vi "Bounce Window_Log In.vi"(8 "Error in":errorcluster, 11 "User Account Table Path":path) -> (0 "Error Out":errorcluster, 3 "User Account Data Out":T1={"帳號 :"="", "權限等級："=enum."開發人員", "建立時間："="", "修改時間："="", "到期時間："="", "狀態："=enum."可使用", "期限："=enum."一天", "密碼："=""})   [LabVIEW 2015]
uses:
  <vilib>/Utility/miscctls.llb/LVPointTypeDef.ctl
panel:
  in  "取消":bool
  in  "登入":bool
  in  "密碼 :":string
  in  "帳號 :":string
  # "帳號登入"
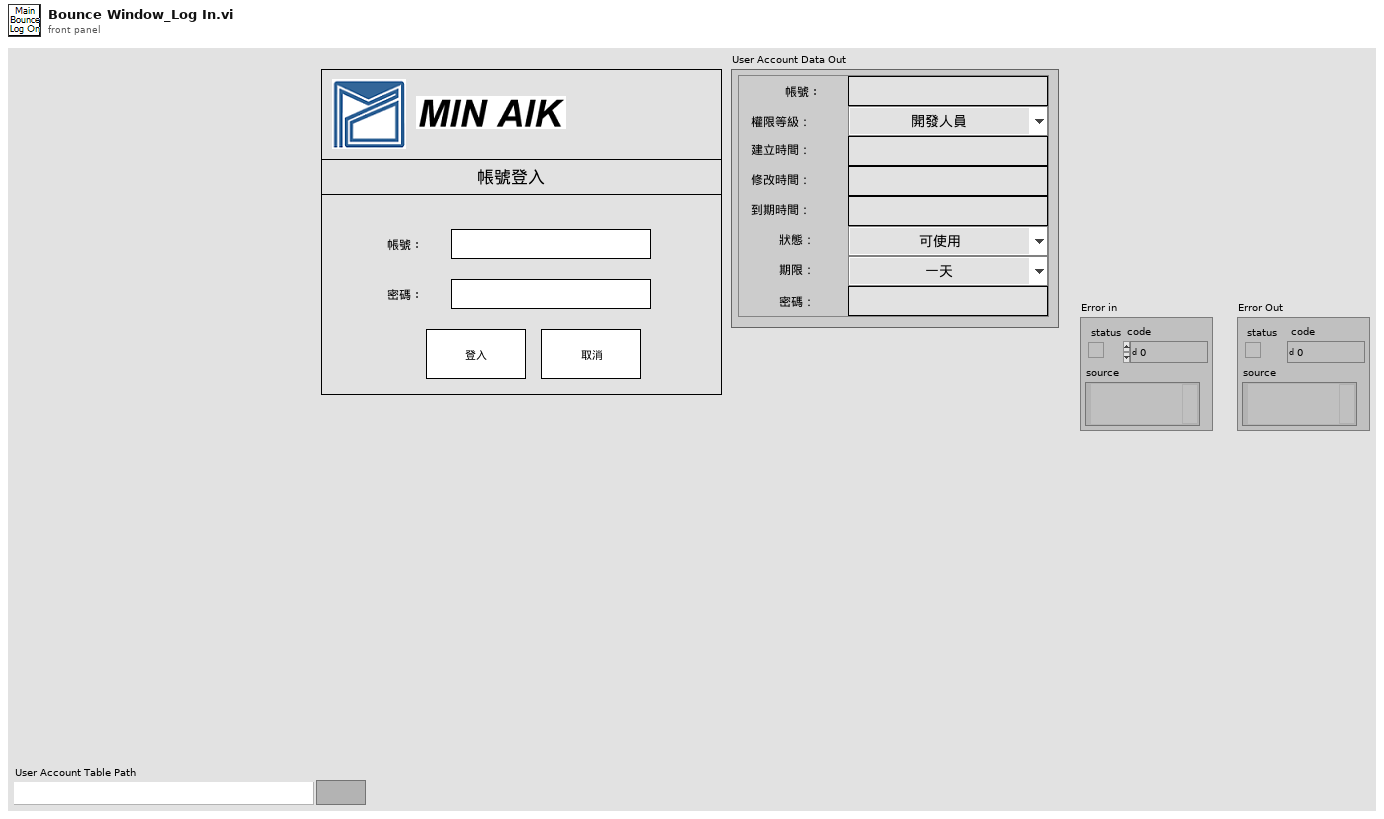
[diagram p1: front panel]
types:
  T1 = typedef "Control_User account_Data.ctl" = cluster{"帳號 :":string, "權限等級：":T2, "建立時間：":string, "修改時間：":string, "到期時間：":string, "狀態：":T3, "期限：":T4, "密碼：":string}
  T2 = typedef "Control_User account_Permissions.ctl" = enum16{"開發人員", "管理者", "工程師", "作業員"}
  T3 = typedef "Control_User Accounts_Status.ctl" = enum16{"可使用", "不可使用"}
  T4 = typedef "Control_User account_Date.ctl" = enum16{"零天", "一天", "七天", "一個月", "一年", "三年"}
  T5 = typedef "Control_Bounce Window_User Accounts_Data Action" = enum16{"Initialize", "Set Data", "Set Data Array", "Replace Data", "Delete Data", "Get Data", "Get Data Array"}
  T6 = typedef "LVPointTypeDef.ctl" = cluster{"Horizontal":i16, "Vertical":i16}
  T7 = typedef "eventvkey.ctl" = enum16{"ASCII", "Enter", "Return", "Shift", "Ctrl", "Alt", "Cmd", "Opt", "Caps", "NumLock", "Clear", "Break", "Up", "Down", "Left", "Right", "Insert", "Delete", "Home", "End", "PageUp", "PageDown", "Escape", "Help", "Pause", "ScrollLock", "F1", "F2", "F3", "F4", "F5", "F6", "F7", "F8", "F9", "F10", "F11", "F12", "F13", "F14", "F15", "F16", "F17", "F18", "F19", "F20", "F21", "F22", "F23", "F24", "Play", "VolumeUp", "VolumeDown", "Mute", "Two Byte Char"}
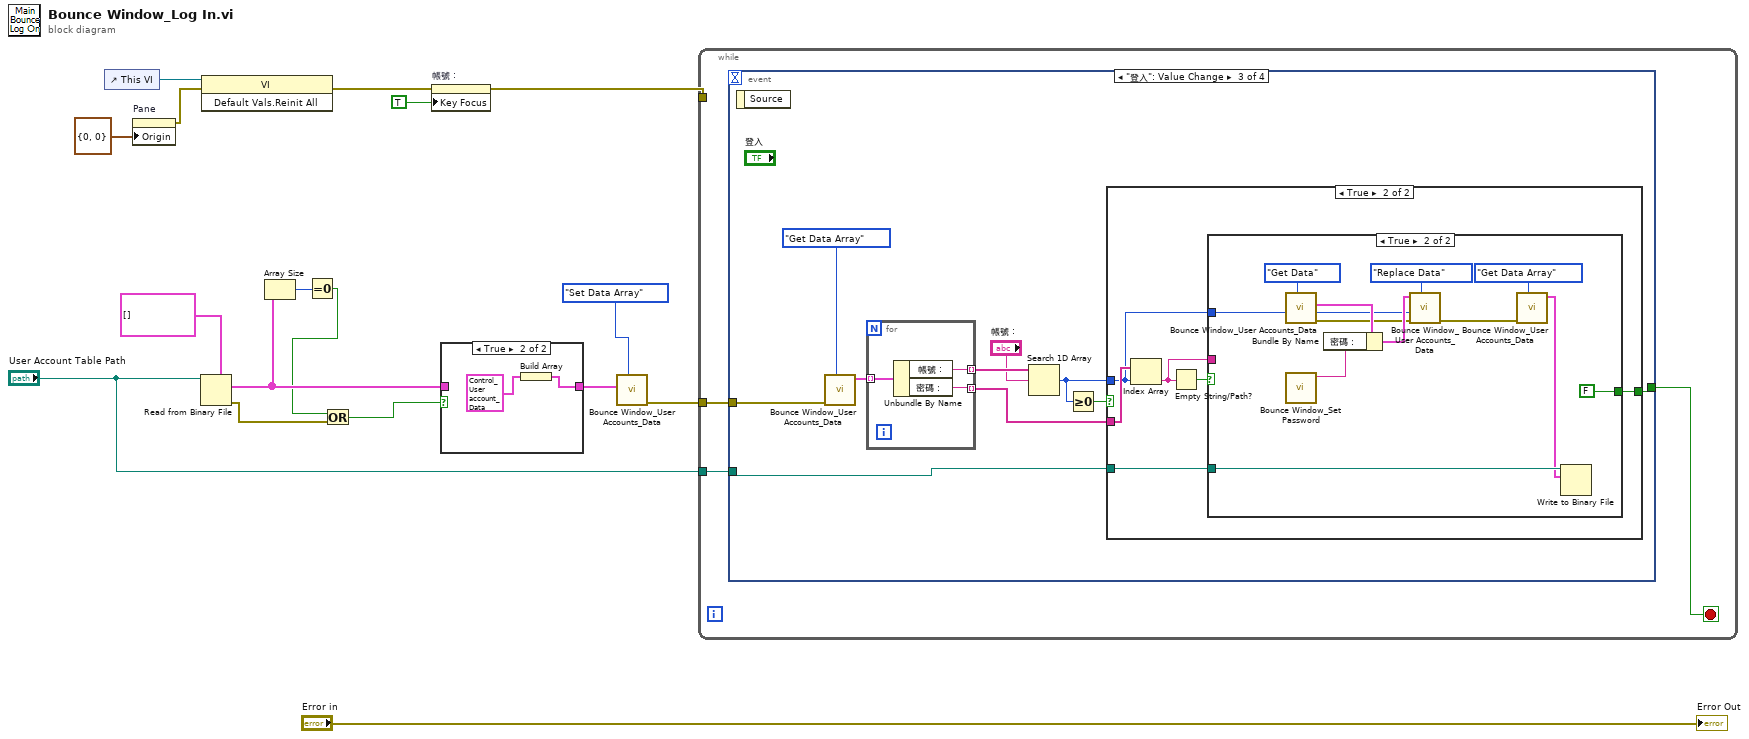
[diagram p0: block diagram]
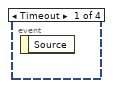
[diagram p3: hidden frame]
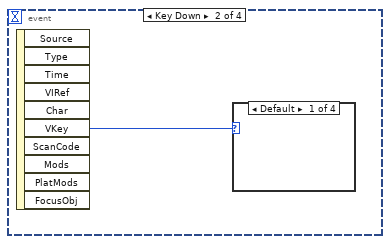
[diagram p4: hidden frame]
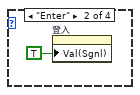
[diagram p5: hidden frame]
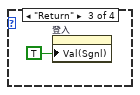
[diagram p6: hidden frame]
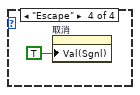
[diagram p7: hidden frame]
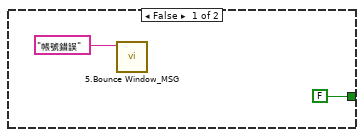
[diagram p8: hidden frame]
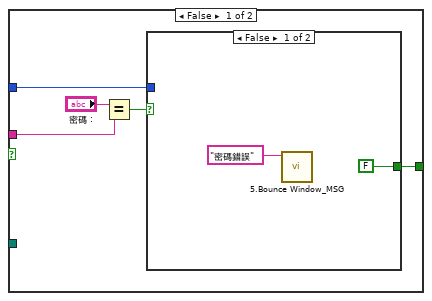
[diagram p9: hidden frame]
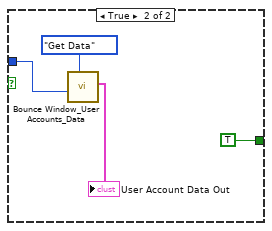
[diagram p10: hidden frame]
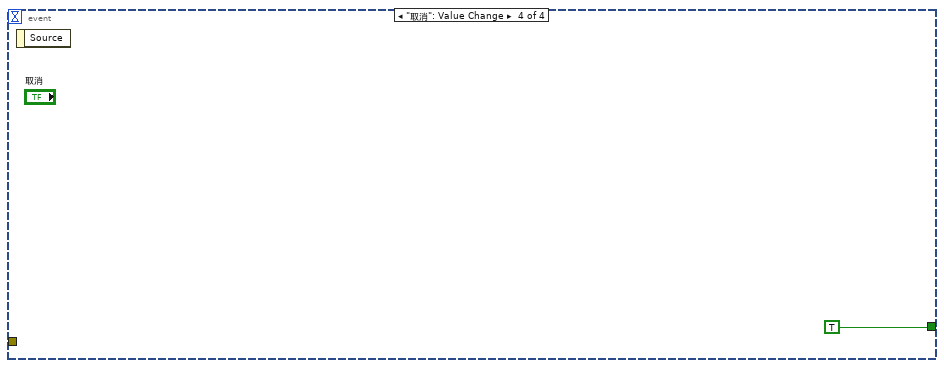
[diagram p11: hidden frame]
diagram:
  n1 = control-ref of="This VI"() -> (w9:refnum<vi>)
  n2 = property on="Pane" class="Pane"("Origin"=T6 {"Horizontal"=0, "Vertical"=0}) -> (error out=w8:errorcluster)  [unwired: 2 in, 1 out]
  n3 = Read from Binary File(5:T1[] [], 11:"User Account Table Path") -> (0:w2:errorcluster, 2:w5:T1[])  [unwired: 4 in, 2 out]
  n4 = invoke class="VI" method="Default Vals.Reinit All"(reference=w9, error in=w8) -> (error out=w11:errorcluster)  [unwired: 1 in, 2 out]
  n5 = Array Size(array=w5) -> (size(s)=w4:i32)
  n6 = Equal To 0?(x=w4) -> (x = 0?=w3:bool)
  n7 = Or(x=w3, y=w2) -> (x .or. y?=w1:bool)
  n8 = property on="帳號 :" class="Str"(error in=w11, "Key Focus"=TRUE) -> (error out=w10:errorcluster)  [unwired: 1 in, 1 out]
  n9 = case shown="True" w1 {
    tunnel: w5 -> [w18 _]
    tunnel: [w18 w19] -> w7
    frame False {
    }
    frame True {
      n10 = Build Array(T1 {"帳號 :"="admin", "權限等級："=enum."開發人員", "建立時間："="2000/01/01", "修改時間："="", "到期時間："="9999/12/31", "狀態："=enum."可使用", "期限："=enum."三年", "密碼："="1234"} ("User Account Data")) -> (w19:T1[])
    }
  }
  n11 = call "Bounce Window_User Accounts_Data.vi"("Table_Action"=Control_Bounce_Window_User_Accounts_Data_Action."Set Data Array", "Data Array In"=w7) -> ("Error Out"=w13:errorcluster)  [unwired: 7 in, 2 out]
  n12 = while {
    tunnel: "User Account Table Path" -> [w22]
    tunnel: w13 -> [w21]
    tunnel: w10 -> [_]
    stop <- w23 stop-if-true
    n13 = event shown="[2] \"登入\": Value Change" {
      selector: _ -> [_ _ _ _]
      dyn-events: _ -> [_ _ _ _]
      timeout: _ -> [_ _ _ _]
      tunnel: [_ _ w32 TRUE] -> w23
      tunnel: w22 -> [_ _ w31 _]
      tunnel: w21 -> [_ _ w28 _]
      event Timeout {
        n14 = event-data() -> ()  [unwired: 1 in, 1 out]
      }
      event Key Down {
        n15 = event-data() -> ("VKey"=w24:T7)  [unwired: 1 in, 9 out]
        n16 = case shown="Default" w24 {
          frame Default {
          }
          frame "Enter" {
            n17 = property on="登入" class="Bool (strict)"("Val(Sgnl)"=TRUE ("Value (Signaling)")) -> ()  [unwired: 2 in, 2 out]
          }
          frame "Return" {
            n18 = property on="登入" class="Bool (strict)"("Val(Sgnl)"=TRUE ("Value (Signaling)")) -> ()  [unwired: 2 in, 2 out]
          }
          frame "Escape" {
            n19 = property on="取消" class="Bool (strict)"("Val(Sgnl)"=TRUE ("Value (Signaling)")) -> ()  [unwired: 2 in, 2 out]
          }
        }
      }
      event "登入": Value Change {
        n20 = event-data() -> ()  [unwired: 1 in, 1 out]
        n21 = call "Bounce Window_User Accounts_Data.vi"("Table_Action"=Control_Bounce_Window_User_Accounts_Data_Action."Get Data Array", "Error in"=w28) -> ("Data Array Out"=w29:T1[])  [unwired: 7 in, 2 out]
        n22 = for {
          tunnel: w29 -> [w71] mode=indexing
          tunnel: [w70] -> w37 mode=indexing
          tunnel: [w69] -> w33 mode=indexing
          n23 = Unbundle By Name(w71) -> ("帳號 :"=w70:string, "密碼："=w69:string)
        }
        n24 = Search 1D Array(1D array=w37, element="帳號 :") -> (index of element=w34:i32)  [unwired: 1 in]
        n25 = Greater Or Equal To 0?(x=w34) -> (x >= 0?=w35:bool)
        n26 = case shown="True" w35 {
          tunnel: w34 -> [_ w41]
          tunnel: w33 -> [_ w45]
          tunnel: [FALSE w42] -> w32
          tunnel: w31 -> [_ w40]
          frame False {
            n27 = call "5.Bounce Window_MSG.vi"("MSG In"="帳號錯誤" ("message")) -> ()  [unwired: 11 in]
          }
          frame True {
            n28 = Index Array(array=w45, index=w41) -> (element=w43:string)
            n29 = Empty String/Path?(string/path=w43) -> (empty?=w44:bool)
            n30 = case shown="True" w44 {
              tunnel: w43 -> [w49 _]
              tunnel: [w47 FALSE] -> w42
              tunnel: w41 -> [w46 w63]
              tunnel: w40 -> [_ w58]
              frame False {
                n31 = Equal?(x="密碼 :", y=w49) -> (x = y?=w48:bool)
                n32 = case shown="False" w48 {
                  tunnel: [FALSE TRUE] -> w47
                  tunnel: w46 -> [_ w54]
                  frame False {
                    n33 = call "5.Bounce Window_MSG.vi"("MSG In"="密碼錯誤" ("message")) -> ()  [unwired: 11 in]
                  }
                  frame True {
                    n34 = call "Bounce Window_User Accounts_Data.vi"("Table_Action"=Control_Bounce_Window_User_Accounts_Data_Action."Get Data", "Row"=w54) -> ("User Account Data Out"=→"User Account Data Out":T1)  [unwired: 7 in, 2 out]
                  }
                }
              }
              frame True {
                n35 = call "Bounce Window_User Accounts_Data.vi"("Table_Action"=Control_Bounce_Window_User_Accounts_Data_Action."Get Data", "Row"=w63) -> ("Error Out"=w61:errorcluster, "User Account Data Out"=w65:T1)  [unwired: 7 in, 1 out]
                n36 = call "Bounce Window_Set Password.vi"() -> ("新密碼 Out"=w62:string)  [unwired: 11 in]
                n37 = Bundle By Name(cluster=w65, "密碼："=w62) -> (w64:T1)
                n38 = call "Bounce Window_User Accounts_Data.vi"("Table_Action"=Control_Bounce_Window_User_Accounts_Data_Action."Replace Data", "Error in"=w61, "Row"=w63, "User Account Data In"=w64) -> ("Error Out"=w60:errorcluster)  [unwired: 5 in, 2 out]
                n39 = call "Bounce Window_User Accounts_Data.vi"("Table_Action"=Control_Bounce_Window_User_Accounts_Data_Action."Get Data Array", "Error in"=w60) -> ("Data Array Out"=w57:T1[])  [unwired: 7 in, 2 out]
                n40 = Write to Binary File(file (use dialog)=w58, data=w57) -> ()  [unwired: 4 in, 3 out]
              }
            }
          }
        }
      }
      event "取消": Value Change {
        n41 = event-data() -> ()  [unwired: 1 in, 1 out]
      }
    }
  }
  "Error Out" <- "Error in"
